vi "Digital Write.vi"   [LabVIEW 2014, in "LMH-LINX.lvlib"]
doc: "Write value(s) to the specified digital output channel(s)."
uses:
  <vilib>/MakerHub/LINX/LMH-LINX.lvlib
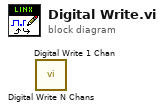
[diagram p0: block diagram]
diagram:
  n1 = call <vilib>:"Digital Write N Chans.vi"() -> ()  [unwired: 10 in, 2 out]
  n2 = call <vilib>:"Digital Write 1 Chan.vi"() -> ()  [unwired: 10 in, 2 out]
